vi "Set chucks on or off.vi"(8 "error in":errorcluster, 10 "Populated on/off":bool=TRUE, 11 "Chuck Control ref in":T1) -> (0 "error out":errorcluster, 3 "Chuck Control ref out":T1)   [LabVIEW 2011]
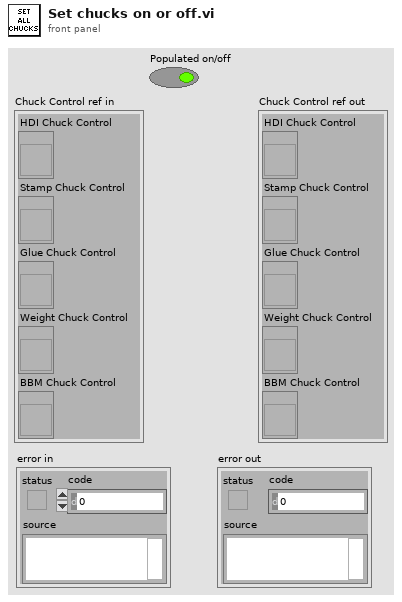
[diagram p1: front panel]
types:
  T1 = cluster{"HDI Chuck Control":refnum<vi>, "Stamp Chuck Control":refnum<vi>, "Glue Chuck Control":refnum<vi>, "Weight Chuck Control":refnum<vi>, "BBM Chuck Control":refnum<vi>}
  T2 = typedef "HDI Chuck Control.ctl" = cluster{"Slot 1":T3, "Slot 2":T3, "Slot 3":T3, "Slot 4":T3}
  T3 = typedef "HDI Slot Control.ctl" = cluster{"Populated?":bool, "Identification:":string}
  T4 = typedef "Glue Chuck Control.ctl" = cluster{"Slot 1":T5, "Slot 2":T5, "Slot 3":T5, "Slot 4":T5}
  T5 = typedef "Glue Slot Control.ctl" = cluster{"Populated?":bool}
  T6 = typedef "Stamp Chuck Control.ctl" = cluster{"Slot 1":T7, "Slot 2":T7, "Slot 3":T7, "Slot 4":T7}
  T7 = typedef "Stamp Slot Control.ctl" = cluster{"Populated?":bool, "Stamp Type":T8}
  T8 = typedef "Stamp Type.ctl" = enum16{"Stamp 1", "Stamp 2", "Stamp 3", "Stamp 4", "Stamp 5", "Stamp 6", "Stamp 7", "Stamp 8"}
  T9 = typedef "Weight Chuck Control.ctl" = cluster{"Slot 1":T10, "Slot 2":T10, "Slot 3":T10, "Slot 4":T10}
  T10 = typedef "Weight Slot Control.ctl" = cluster{"Populated?":bool, "Weight Type":T11}
  T11 = typedef "Weight Type.ctl" = enum16{"Weight 1", "Weight 2", "Weight 3", "Weight 4", "Weight 5", "Weight 6", "Weight 7", "Weight 8", "Weight 9", "Weight 10", "Weight 11", "Weight 12", "Weight 13", "Weight 14", "Weight 15", "Weight 16"}
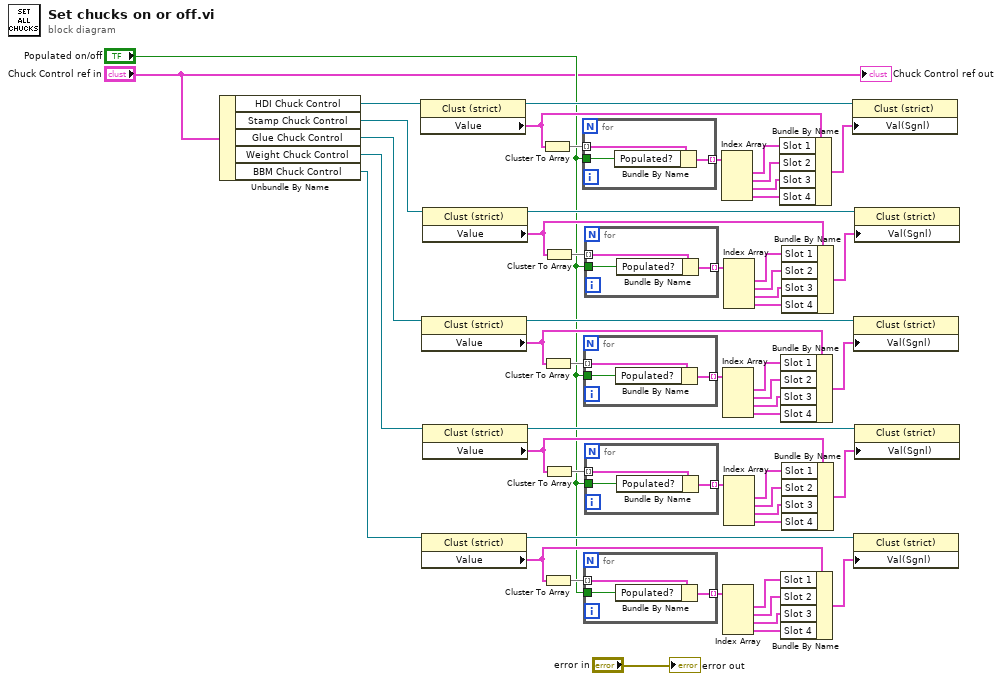
[diagram p0: block diagram]
diagram:
  n1 = Unbundle By Name("Chuck Control ref in") -> ("HDI Chuck Control"=w45:refnum<vi>, "Stamp Chuck Control"=w25:refnum<vi>, "Glue Chuck Control"=w24:refnum<vi>, "Weight Chuck Control"=w4:refnum<vi>, "BBM Chuck Control"=w3:refnum<vi>)
  n2 = property class="Clust (strict)"(reference=w45) -> (reference out=w44:refnum<vi>, "Value"=w46:T2)  [unwired: 1 in, 1 out]
  n3 = property class="Clust (strict)"(reference=w24) -> (reference out=w26:refnum<vi>, "Value"=w27:T4)  [unwired: 1 in, 1 out]
  n4 = property class="Clust (strict)"(reference=w3) -> (reference out=w6:refnum<vi>, "Value"=w7:T2)  [unwired: 1 in, 1 out]
  n5 = property class="Clust (strict)"(reference=w25) -> (reference out=w35:refnum<vi>, "Value"=w36:T6)  [unwired: 1 in, 1 out]
  n6 = property class="Clust (strict)"(reference=w4) -> (reference out=w15:refnum<vi>, "Value"=w16:T9)  [unwired: 1 in, 1 out]
  n7 = Cluster To Array(cluster=w46) -> (array=w47:T3[])
  n8 = Cluster To Array(cluster=w27) -> (array=w28:T5[])
  n9 = Cluster To Array(cluster=w7) -> (array=w8:T3[])
  n10 = Cluster To Array(cluster=w36) -> (array=w37:T7[])
  n11 = Cluster To Array(cluster=w16) -> (array=w17:T10[])
  n12 = for {
    tunnel: [w56] -> w52 mode=indexing
    tunnel: w47 -> [w55] mode=indexing
    tunnel: "Populated on/off" -> [w54]
    n13 = Bundle By Name(cluster=w55, "Populated?"=w54) -> (w56:T3)
  }
  n14 = for {
    tunnel: [w59] -> w33 mode=indexing
    tunnel: w28 -> [w58] mode=indexing
    tunnel: "Populated on/off" -> [w57]
    n15 = Bundle By Name(cluster=w58, "Populated?"=w57) -> (w59:T5)
  }
  n16 = for {
    tunnel: [w62] -> w13 mode=indexing
    tunnel: w8 -> [w61] mode=indexing
    tunnel: "Populated on/off" -> [w60]
    n17 = Bundle By Name(cluster=w61, "Populated?"=w60) -> (w62:T3)
  }
  n18 = for {
    tunnel: [w65] -> w42 mode=indexing
    tunnel: w37 -> [w64] mode=indexing
    tunnel: "Populated on/off" -> [w63]
    n19 = Bundle By Name(cluster=w64, "Populated?"=w63) -> (w65:T7)
  }
  n20 = for {
    tunnel: [w68] -> w22 mode=indexing
    tunnel: w17 -> [w67] mode=indexing
    tunnel: "Populated on/off" -> [w66]
    n21 = Bundle By Name(cluster=w67, "Populated?"=w66) -> (w68:T10)
  }
  n22 = Index Array(array=w52) -> (element #1=w51:T3, element #2=w50:T3, element #3=w49:T3, element #4=w48:T3)  [unwired: 4 in]
  n23 = Index Array(array=w33) -> (element #1=w32:T5, element #2=w31:T5, element #3=w30:T5, element #4=w29:T5)  [unwired: 4 in]
  n24 = Index Array(array=w13) -> (element #1=w12:T3, element #2=w11:T3, element #3=w10:T3, element #4=w9:T3)  [unwired: 4 in]
  n25 = Index Array(array=w42) -> (element #1=w41:T7, element #2=w40:T7, element #3=w39:T7, element #4=w38:T7)  [unwired: 4 in]
  n26 = Index Array(array=w22) -> (element #1=w21:T10, element #2=w20:T10, element #3=w19:T10, element #4=w18:T10)  [unwired: 4 in]
  n27 = Bundle By Name(cluster=w46, "Slot 1"=w51, "Slot 2"=w50, "Slot 3"=w49, "Slot 4"=w48) -> (w53:T2)
  n28 = Bundle By Name(cluster=w27, "Slot 1"=w32, "Slot 2"=w31, "Slot 3"=w30, "Slot 4"=w29) -> (w34:T4)
  n29 = Bundle By Name(cluster=w7, "Slot 1"=w12, "Slot 2"=w11, "Slot 3"=w10, "Slot 4"=w9) -> (w14:T2)
  n30 = Bundle By Name(cluster=w36, "Slot 1"=w41, "Slot 2"=w40, "Slot 3"=w39, "Slot 4"=w38) -> (w43:T6)
  n31 = Bundle By Name(cluster=w16, "Slot 1"=w21, "Slot 2"=w20, "Slot 3"=w19, "Slot 4"=w18) -> (w23:T9)
  n32 = property class="Clust (strict)"(reference=w44, "Val(Sgnl)"=w53) -> ()  [unwired: 1 in, 2 out]
  n33 = property class="Clust (strict)"(reference=w26, "Val(Sgnl)"=w34) -> ()  [unwired: 1 in, 2 out]
  n34 = property class="Clust (strict)"(reference=w6, "Val(Sgnl)"=w14) -> ()  [unwired: 1 in, 2 out]
  n35 = property class="Clust (strict)"(reference=w35, "Val(Sgnl)"=w43) -> ()  [unwired: 1 in, 2 out]
  n36 = property class="Clust (strict)"(reference=w15, "Val(Sgnl)"=w23) -> ()  [unwired: 1 in, 2 out]
  "error out" <- "error in"
  "Chuck Control ref out" <- "Chuck Control ref in"
